vi "MeasurementConfig.vi"() -> (2 "Array 2":T1(array[cluster]))   [LabVIEW 2019]
uses:
  Components/MeasurementConfigGlobals.vi
panel:
  in  "Array":T1(array[cluster])
  in  "Name":string
  in  "OK Button":bool
  in  "Address":refnum<visa-resource-name>
  in  "Clear":bool
  in  "Freq/Delay":dbl
  in  "Measurment Type":string(combo)
  in  "I Max":dbl
  in  "Add Measurement":bool
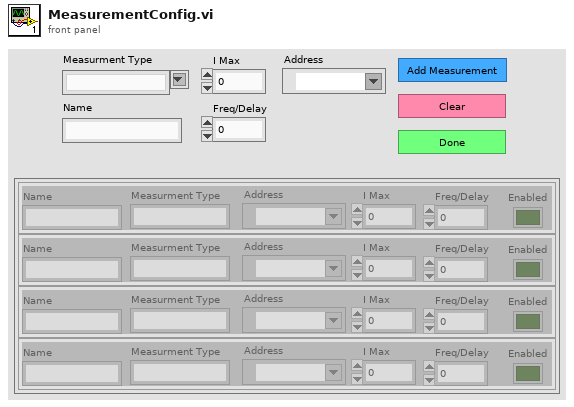
[diagram p1: front panel]
types:
  T1 = cluster{"Name":string, "Measurment Type":string, "I Max":dbl, "Freq/Delay":dbl, "Address":refnum<visa-resource-name>, "Enabled":bool}[]
  T2 = cluster{"Name":string, "Measurment Type":string, "I Max":dbl, "Freq/Delay":dbl, "Address":refnum<visa-resource-name>, "Enabled":bool}
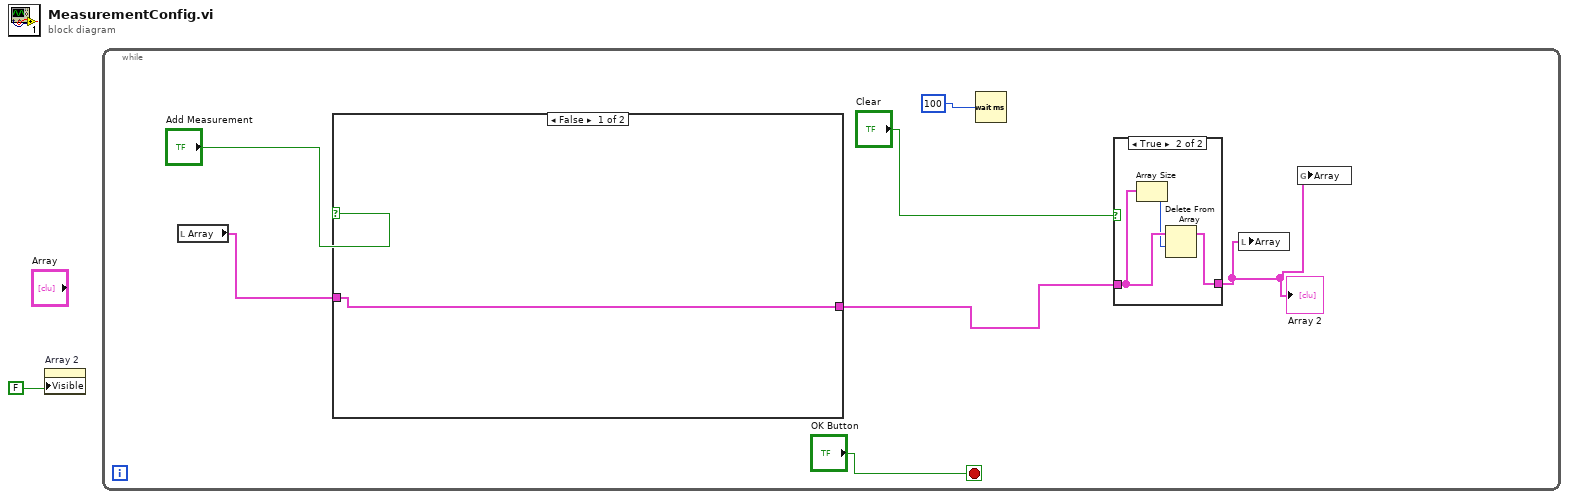
[diagram p0: block diagram]
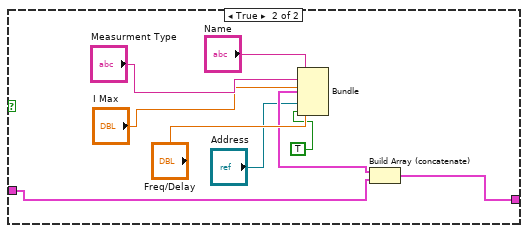
[diagram p3: hidden frame]
diagram:
  n1 = property on="Array 2" class="Arr (strict)"("Visible"=FALSE) -> ()  [unwired: 2 in, 2 out]
  n2 = while {
    stop <- "OK Button" stop-if-true
    n3 = local read "Array"() -> (w4:T1)
    n4 = case shown="False" "Add Measurement" {
      tunnel: [w13 w22] -> w6
      tunnel: w4 -> [w13 w14]
      frame False {
      }
      frame True {
        n5 = Bundle("Name"="Name", "Measurment Type"="Measurment Type", "I Max"="I Max", "Freq/Delay"="Freq/Delay", "Address"="Address", "Enabled"=TRUE) -> (w18:T2)  [unwired: 1 in]
        n6 = Build Array (concatenate)(w18, w14) -> (w22:T1)
      }
    }
    n7 = Wait (ms)(milliseconds to wait=100) -> ()  [unwired: 1 out]
    n8 = case shown="True" "Clear" {
      tunnel: w6 -> [w9 w11]
      tunnel: [w9 w12] -> w2
      frame False {
      }
      frame True {
        n9 = Array Size(array=w11) -> (size(s)=w10:i32)
        n10 = Delete From Array(array=w11, length=w10) -> (array with subset deleted=w12:T1)  [unwired: 1 in, 1 out]
      }
    }
    "Array 2" <- w2
    n11 = local write "Array"(w2) -> ()
    n12 = global write "MeasurementConfigGlobals.vi" "Array"(w2) -> ()
  }
